vi "time_gmtsec.vi"(2 "Timezone Offset (Hrs)":i32=5, 3 "Timestamp":timestamp) -> (0 "Fractional Sec Since 12AM GMT":dbl, 1 "Sec Since 12AM GMT":u32)   [LabVIEW 2018]
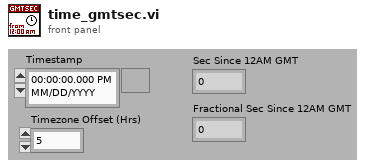
[diagram p1: front panel]
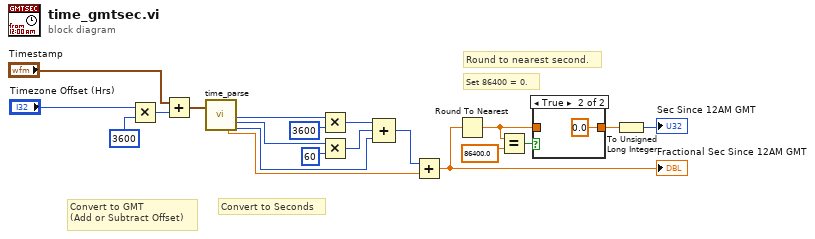
[diagram p0: block diagram]
diagram:
  # "Set 86400 = 0."
  # "Round to nearest second."
  # "Convert to Seconds"
  # "Convert to GMT\n(Add or Subtract Offset)"
  n1 = Multiply(x="Timezone Offset (Hrs)", y=3600) -> (x*y=w14:i32)
  n2 = Add(x="Timestamp", y=w14) -> (x+y=w16:timestamp)
  n3 = call "time_parse.vi"("Current Time"=w16) -> ("Fractional Seconds"=w8:dbl, "Hour"=w20:u32, "Minutes"=w19:u32, "Seconds"=w11:u32)  [unwired: 12 in, 3 out]
  n4 = Multiply(x=w20, y=u32 3600) -> (x*y=w9:u32)
  n5 = Multiply(x=w19, y=u32 60) -> (x*y=w10:u32)
  n6 = Compound Arithmetic op=ADD(w9, w10, w11) -> (w7:u32)
  n7 = Add(x=w7, y=w8) -> (x+y=w3:dbl)
  "Fractional Sec Since 12AM GMT" <- w3
  n8 = Round To Nearest(number=w3) -> (nearest integer value=w4:dbl)
  n9 = Equal?(x=w4, y=86400.0) -> (x = y?=w6:bool)
  n10 = case shown="True" w6 {
    tunnel: [w21 0.0] -> w2
    tunnel: w4 -> [w21 _]
    frame False {
    }
    frame True {
    }
  }
  n11 = To Unsigned Long Integer(number=w2) -> (unsigned 32bit integer=→"Sec Since 12AM GMT":u32)
